vi "excelChart.vi"() -> ()   [LabVIEW 2012]
uses:
  <vilib>/Utility/NIReport.llb/Generate Report Object Reference.ctl
  <vilib>/Utility/NIReport.llb/NI_report.lvclass
  <vilib>/addons/database/Auxilliary.llb/DB Tools Cursor Type.ctl
  <vilib>/addons/database/Connection.llb/DB Tools Open Connec (Path).vi
  <vilib>/addons/database/Connection.llb/Conn Execute.vi
  <vilib>/addons/database/Recordset.llb/Rec Fetch Recordset Data (R).vi
  <vilib>/addons/database/Recordset.llb/Rec Destroy - Connection.vi
  <vilib>/Utility/NIReport.llb/Append Text Table to Report (wrap).vi
  <vilib>/addons/database/_DB Variant To Data/Database Variant To Data.xnode
  <vilib>/addons/database/NI_Database_API.lvlib
  <vilib>/Utility/NIReport.llb/Excel/NI_Excel.lvclass
  <vilib>/addons/_office/NI_ReportGenerationToolkit.lvlib
panel:
  in  "Running":string[][](table)
  in  "Report Template":path=path "E:/m100/data/AT.xls"
  out "report out":T1
  out "error out":errorcluster
  out "Row Headers":string[](array[string])
  in  "From Date":string="2014/9/20"
  in  "End Date":string="2014/9/24"
  in  "Shift":string(combo)
  in  "customer":string
  in  "device":string
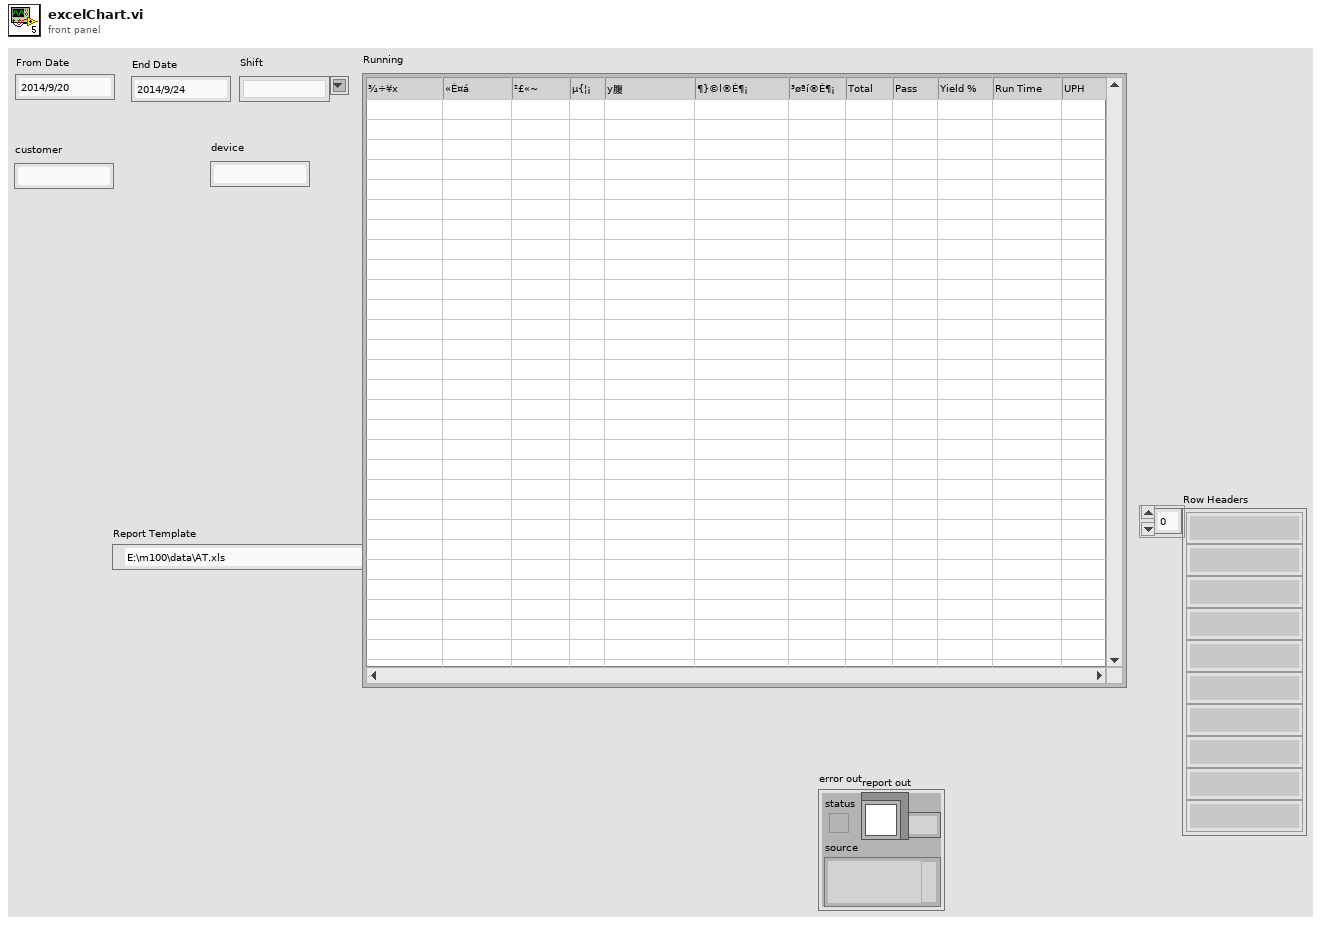
[diagram p1: front panel]
types:
  T1 = typedef "Generate Report Object Reference.ctl" = refnum<class "NI_report.lvclass">
  T2 = typedef "NI_Database_API.lvlib/DB Tools Cursor Type.ctl" = enum16{"forward-only", "keyset", "dynamic", "static"}
  T3 = typedef "NI_Database_API.lvlib/Conn ObjectReference.ctl" = refnum<k1>
  T4 = typedef "NI_Database_API.lvlib/Rec ObjectReference.ctl" = refnum<k1>
  T5 = enum16{"Standard Report", "HTML", "Word", "Excel"}
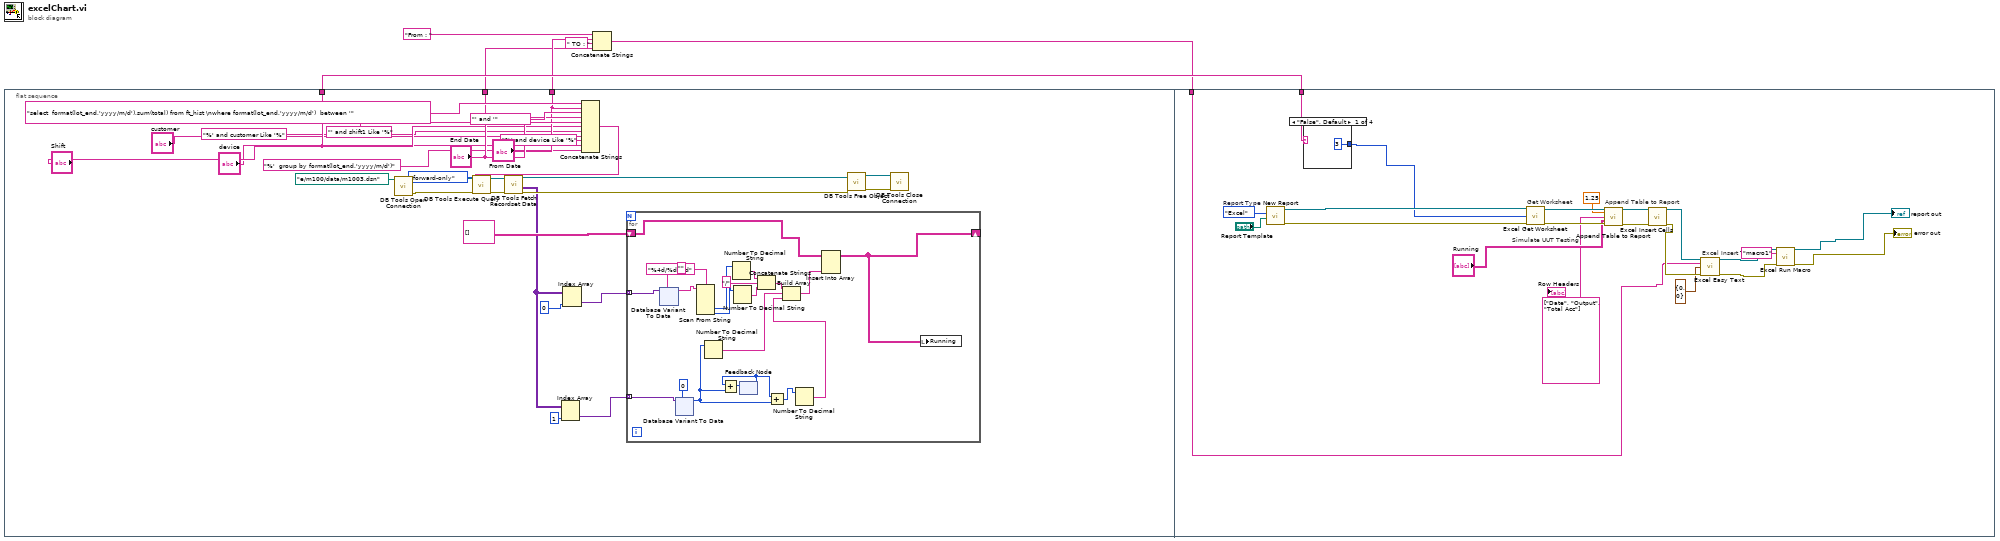
[diagram p0: block diagram]
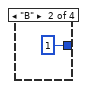
[diagram p2: hidden frame]
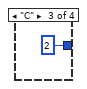
[diagram p3: hidden frame]
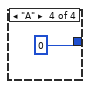
[diagram p4: hidden frame]
diagram:
  n1 = flat-sequence {
    tunnel: ["Shift"] -> w6
    tunnel: ["From Date"] -> w4
    tunnel: ["End Date"] -> w2
    tunnel: w6 -> [w128]
    tunnel: w1 -> [w126]
    frame #0 {
      n2 = call-poly <vilib>:"DB Tools Open Connection.vi"("connection information"=path "e:/m100/data/m1003.dsn") -> ("error out"=w22:errorcluster, "connection reference"=w23:T3)  [unwired: 7 in]
      n3 = Concatenate Strings("select  format(lot_end,'yyyy/m/d'),sum(total) from ft_hist \nwhere format(lot_end,'yyyy/m/d')  between '" ("string"), "From Date", "' and '" ("string"), "End Date", "' and shift1 Like '%" ("string"), "Shift", "%' and customer Like '%" ("string"), "customer", "%' and device Like '%" ("string"), "device", "%'  group by format(lot_end,'yyyy/m/d')" ("string")) -> (w19:string)
      n4 = call-poly <vilib>:"DB Tools Execute Query.vi"("error in (no error)"=w22, "cursor type"=DB_Tools_Cursor_Type."forward-only", "SQL query"=w19, "connection reference"=w23) -> ("error out"=w25:errorcluster, "recordset reference"=w24:T4)  [unwired: 4 in]
      n5 = call-poly <vilib>:"DB Tools Fetch Recordset Data.vi"("error in (no error)"=w25, "recordset reference"=w24) -> ("error out"=w21:errorcluster, "recordset data"=w12:variant[][], "recordset reference out"=w20:T4)  [unwired: 3 in]
      n6 = Index Array(array=w12, index (col)=1) -> (element=w31:variant[])  [unwired: 1 in]
      n7 = Index Array(array=w12, index (col)=0) -> (element=w29:variant[])  [unwired: 1 in]
      n8 = for {
        shift-right: [w35] -> _
        shift-left: string[][] [] -> [w37]
        tunnel: w31 -> [w55] mode=indexing
        tunnel: w29 -> [w54] mode=indexing
        n9 = xnode "Database Variant To Data"("database variant"=w54, "type"="") -> ("data"=w50:string)  [unwired: 1 in, 1 out]
        n10 = xnode "Database Variant To Data"("database variant"=w55, "type"=0) -> ("data"=w40:i32)  [unwired: 1 in, 1 out]
        n11 = Scan From String(format string="%4d/%d/%d", input string=w50) -> (output 2=w48:i32, output 3=w47:i32)  [unwired: 6 in, 3 out]
        n12 = Number To Decimal String(number=w40) -> (decimal integer string=w53:string)  [unwired: 1 in]
        n13 = Number To Decimal String(number=w48) -> (decimal integer string=w46:string)  [unwired: 1 in]
        n14 = Number To Decimal String(number=w47) -> (decimal integer string=w44:string)  [unwired: 1 in]
        n15 = feedback #1() -> (w41:i32)  [unwired: 1 in]
        n16 = Add(x=w41, y=w40) -> (x+y=w42:i32)
        n17 = feedback-in #1(w42) -> ()
        n18 = Concatenate Strings(w46, "/" ("string"), w44) -> (w43:string)
        n19 = Add(x=w41, y=w40) -> (x+y=w39:i32)
        n20 = Number To Decimal String(number=w39) -> (decimal integer string=w38:string)  [unwired: 1 in]
        n21 = Build Array(w43, w53, w38) -> (w36:string[])
        n22 = Insert Into Array(array=w37, new element=w36) -> (w35:string[][])  [unwired: 2 in]
        n23 = local write "Running"(w35) -> ()
      }
      n24 = call-poly <vilib>:"DB Tools Free Object.vi"("error in (no error)"=w21, "recordset reference"=w20) -> ("error out"=w26:errorcluster, "connection reference"=w27:T3)  [unwired: 8 in]
      n25 = call <vilib>:"DB Tools Close Connection.vi"("error in (no error)"=w26, "connection reference"=w27) -> ()  [unwired: 5 in, 1 out]
    }
    frame #1 {
      w120 = string[] ["Date", "Output", "Total Acc"] ("row headers")
      w141 = T5."Excel"  # Report Type
      # "Excel Insert Text"
      # "Simulate UUT Testing"
      # "Append Table to Report"
      # "Get Worksheet"
      n26 = call <vilib>:"New Report.vi"("report type"=w141, "template (empty)"="Report Template") -> ("report out"=w130:refnum<class "NI_report.lvclass">, "error out"=w129:errorcluster)  [unwired: 12 in]
      n27 = case shown="\"False\", Default" w128 {
        tunnel: [3 1 2 0] -> w127
        frame "False", Default {
        }
        frame "B" {
        }
        frame "C" {
        }
        frame "A" {
        }
      }
      n28 = call <vilib>:"Excel Get Worksheet.vi"("report in"=w130, "worksheet index (0)"=w127, "error in (no error)"=w129) -> ("report out"=w139:refnum<class "NI_report.lvclass">, "error out"=w138:errorcluster)  [unwired: 11 in]
      n29 = call-poly <vilib>:"Append Table to Report.vi"("report in"=w139, "column width (1)"=1.25, "row headers"=w120, "text data"="Running", "error in (no error)"=w138) -> ("report out"=w135:refnum<class "NI_report.lvclass">, "error out"=w134:errorcluster)  [unwired: 7 in, 2 out]
      n30 = call <vilib>:"Excel Insert Cells.vi"("report in"=w135, "error in (no error)"=w134) -> ("report out"=w133:refnum<class "NI_report.lvclass">, "error out"=w132:errorcluster)  [unwired: 12 in]
      n31 = call <vilib>:"Excel Easy Text.vi"("report in"=w133, "text"=w126, "start (-1, -1)"=cluster{"row":i32, "column":i32} {"row"=0, "column"=0} ("end (-1, -1)"), "error in (no error)"=w132) -> ("report out"=w125:refnum<class "NI_report.lvclass">, "error out"=w123:errorcluster)  [unwired: 7 in, 3 out]
      n32 = call <vilib>:"Excel Run Macro.vi"("report in"=w125, "macro name"="macro1", "error in (no error)"=w123) -> ("report out"=→"report out":refnum<class "NI_report.lvclass">, "error out"=→"error out":errorcluster)  [unwired: 10 in, 1 out]
      "Row Headers" <- w120
    }
  }
  n33 = Concatenate Strings("From : " ("string"), w4, " TO : " ("string"), w2) -> (w1:string)
